vi "destroyEvents.vi"(8 "error in (no error)":errorcluster, 11 "MonoPubSubData in":refnum<class "MonoPubSubData.lvclass">) -> (0 "error out":errorcluster, 3 "MonoPubSubData out":refnum<class "MonoPubSubData.lvclass">)   [LabVIEW 2016, in "MonoPubSubData.lvclass"]
uses:
  MonoPubSubData.lvclass
  MonoPubSubData.lvclass/MonoPubSubData.ctl
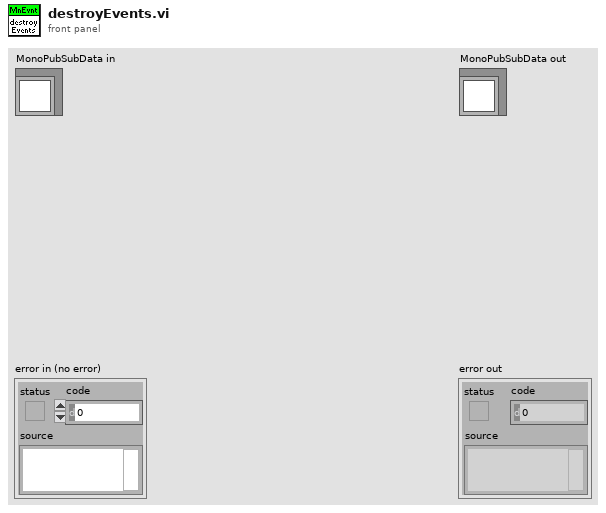
[diagram p1: front panel]
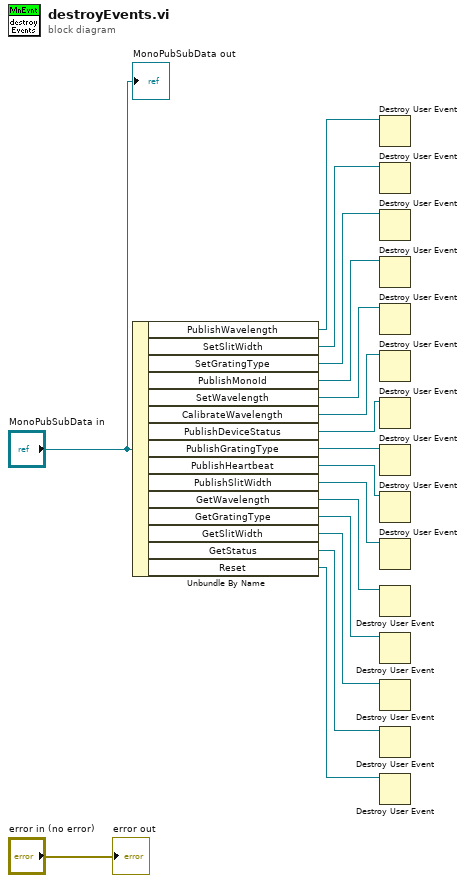
[diagram p0: block diagram]
diagram:
  n1 = Unbundle By Name("MonoPubSubData in") -> ("PublishWavelength"=w15:refnum<user-event>, "SetSlitWidth"=w14:refnum<user-event>, "SetGratingType"=w13:refnum<user-event>, "PublishMonoId"=w12:refnum<user-event>, "SetWavelength"=w11:refnum<user-event>, "CalibrateWavelength"=w10:refnum<user-event>, "PublishDeviceStatus"=w9:refnum<user-event>, "PublishGratingType"=w8:refnum<user-event>, "PublishHeartbeat"=w7:refnum<user-event>, "PublishSlitWidth"=w6:refnum<user-event>, "GetWavelength"=w5:refnum<user-event>, "GetGratingType"=w4:refnum<user-event>, "GetSlitWidth"=w3:refnum<user-event>, "GetStatus"=w2:refnum<user-event>, "Reset"=w1:refnum<user-event>)
  n2 = Destroy User Event(user event=w15) -> ()  [unwired: 1 in, 1 out]
  n3 = Destroy User Event(user event=w14) -> ()  [unwired: 1 in, 1 out]
  n4 = Destroy User Event(user event=w13) -> ()  [unwired: 1 in, 1 out]
  n5 = Destroy User Event(user event=w12) -> ()  [unwired: 1 in, 1 out]
  n6 = Destroy User Event(user event=w11) -> ()  [unwired: 1 in, 1 out]
  n7 = Destroy User Event(user event=w10) -> ()  [unwired: 1 in, 1 out]
  n8 = Destroy User Event(user event=w9) -> ()  [unwired: 1 in, 1 out]
  n9 = Destroy User Event(user event=w8) -> ()  [unwired: 1 in, 1 out]
  n10 = Destroy User Event(user event=w7) -> ()  [unwired: 1 in, 1 out]
  n11 = Destroy User Event(user event=w6) -> ()  [unwired: 1 in, 1 out]
  n12 = Destroy User Event(user event=w5) -> ()  [unwired: 1 in, 1 out]
  n13 = Destroy User Event(user event=w4) -> ()  [unwired: 1 in, 1 out]
  n14 = Destroy User Event(user event=w3) -> ()  [unwired: 1 in, 1 out]
  n15 = Destroy User Event(user event=w2) -> ()  [unwired: 1 in, 1 out]
  n16 = Destroy User Event(user event=w1) -> ()  [unwired: 1 in, 1 out]
  "error out" <- "error in (no error)"
  "MonoPubSubData out" <- "MonoPubSubData in"
